vi "Write2LogFile.vi"(1 "Add to log file":string, 2 "Log file before":string) -> (0 "Log file after":string)   [LabVIEW 2019]
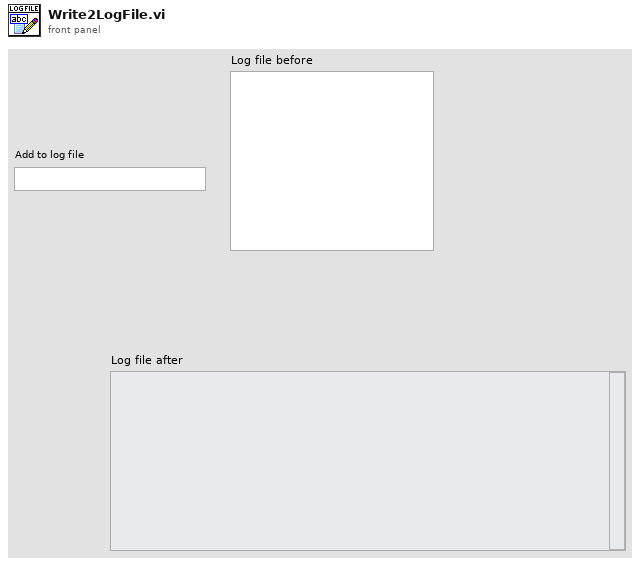
[diagram p1: front panel]
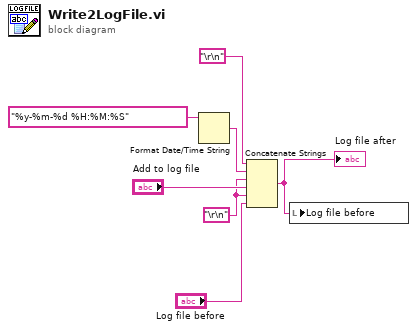
[diagram p0: block diagram]
diagram:
  w3 = "\r\n"
  n1 = Format Date/Time String(time format string (%c)="%y-%m-%d %H:%M:%S") -> (date/time string=w6:string)  [unwired: 2 in]
  n2 = Concatenate Strings("\r\n", w6, w3, "Add to log file", w3, "Log file before") -> (w4:string)
  "Log file after" <- w4
  n3 = local write "Log file before"(w4) -> ()
